vi "Check Status.vi"(8 "error in (no error)":errorcluster, 11 "PEM in":refnum<class "PEM.lvclass">) -> (0 "error out":errorcluster, 1 "Status":string, 2 "Ready?":bool, 3 "PEM out":refnum<class "PEM.lvclass">)   [LabVIEW 2017, in "PEM.lvclass"]
doc: "(Dynamic) Check if the instrument is powered on and update its member fields with the instrument's current status. Optionally return a text status message."
uses:
  PEM.lvclass
  PEM.lvclass/PEM.ctl
  Utility Classes/Scannable/Scannable.lvclass
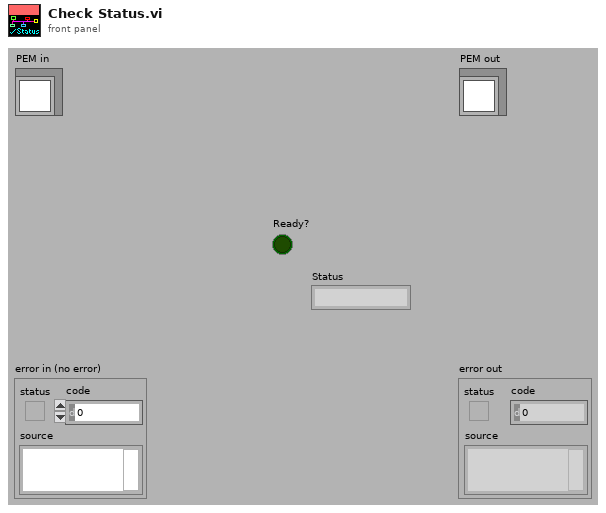
[diagram p1: front panel]
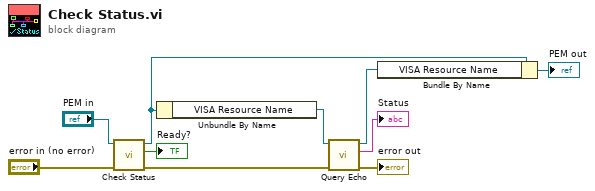
[diagram p0: block diagram]
diagram:
  n1 = call-parent "Check Status.vi"("error in (no error)"="error in (no error)", "Instrument in"="PEM in") -> ("error out"=w2:errorcluster, "Ready?"=→"Ready?":bool, "Instrument out"=w6:refnum<class "PEM.lvclass">)  [unwired: 6 in, 1 out]
  n2 = Unbundle By Name(w6) -> ("VISA Resource Name"=w7:refnum<visa-resource-name>)
  n3 = call "Query Echo.vi"("error in (no error)"=w2, "VISA resource name"=w7) -> ("error out"=→"error out":errorcluster, "Echo output"=→"Status":string, "VISA resource name out"=w8:refnum<visa-resource-name>)  [unwired: 7 in]
  n4 = Bundle By Name(cluster=w6, "VISA Resource Name"=w8) -> (→"PEM out":refnum<class "PEM.lvclass">)
